vi "To Bulleted String.vi"(11 "ProjPath error message":string) -> (3 "String":string)   [LabVIEW 2013, in "TagBusProcessingPluginFeatureDecider.lvclass"]
uses:
  TagBusProcessingPluginFeatureDecider.lvclass
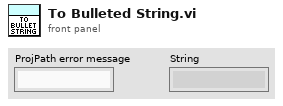
[diagram p1: front panel]
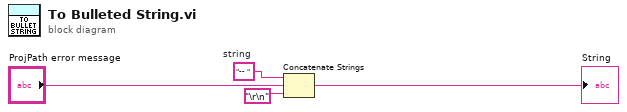
[diagram p0: block diagram]
diagram:
  w2 = "-- "  # string
  n1 = Concatenate Strings(w2, "ProjPath error message", "\r\n") -> (→"String":string)
